vi "AutoRoutineSelector.vi"(4 "NotPurePursuit":bool, 5 "OurSwitch":bool, 6 "RR":dbl, 7 "OurScale":bool, 8 "RL":dbl, 9 "LR":dbl, 10 "LL":dbl, 11 "Position":dbl) -> (3 "File Name":string)   [LabVIEW 2018]
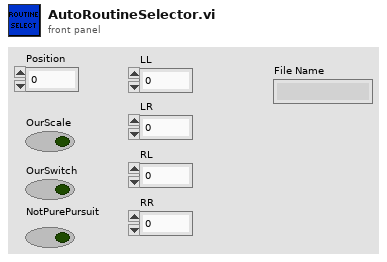
[diagram p1: front panel]
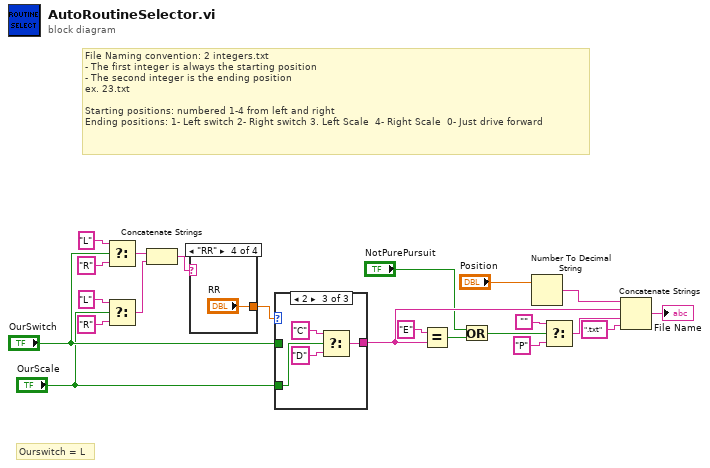
[diagram p0: block diagram]
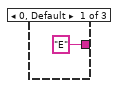
[diagram p2: hidden frame]
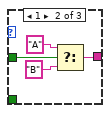
[diagram p3: hidden frame]
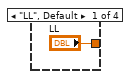
[diagram p4: hidden frame]
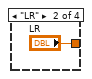
[diagram p5: hidden frame]
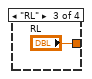
[diagram p6: hidden frame]
diagram:
  # "Ourswitch = L"
  # "File Naming convention: 2 integers.txt \n- The first integer is always the starting position\n- The second integer is the ending position\nex. 23.txt\n\nStarting positions: numbered 1-4 from left and right\nEnding positions: 1- Left switch 2- Right switch 3. Left Scale  4- Right Scale  0- Just drive forward"
  n1 = Select(t="L", s="OurSwitch", f="R") -> (s? t:f=w17:string)
  n2 = Select(t="L", s="OurScale", f="R") -> (s? t:f=w16:string)
  n3 = Concatenate Strings(w17, w16) -> (w15:string)
  n4 = case shown="\"RR\"" w15 {
    tunnel: ["LL" "LR" "RL" "RR"] -> w14
    frame "LL", Default {
    }
    frame "LR" {
    }
    frame "RL" {
    }
    frame "RR" {
    }
  }
  n5 = case shown="2" w14 {
    tunnel: "OurSwitch" -> [_ w29 _]
    tunnel: "OurScale" -> [_ _ w33]
    tunnel: ["E" w28 w32] -> w8
    frame 0, Default {
    }
    frame 1 {
      n6 = Select(t="A", s=w29, f="B") -> (s? t:f=w28:string)
    }
    frame 2 {
      n7 = Select(t="C", s=w33, f="D") -> (s? t:f=w32:string)
    }
  }
  n8 = Equal?(x="E", y=w8) -> (x = y?=w6:bool)
  n9 = Or(x="NotPurePursuit", y=w6) -> (x .or. y?=w4:bool)
  n10 = Number To Decimal String(number="Position") -> (decimal integer string=w10:string)  [unwired: 1 in]
  n11 = Select(t="", s=w4, f="P") -> (s? t:f=w2:string)
  n12 = Concatenate Strings(w10, w8, w2, ".txt") -> (→"File Name":string)
